vi "trigger.vi"(8 "error in (no error)":errorcluster, 11 "handle":u32) -> (0 "error out":errorcluster, 2 "function return":i32, 3 "handle out":i32)   [LabVIEW 2017, in "buddy.lvlib"]
doc: "EXPORT int buddy_trigger(hid_device *handle);"
uses:
  buddy.lvlib
  buddy_x64.dll
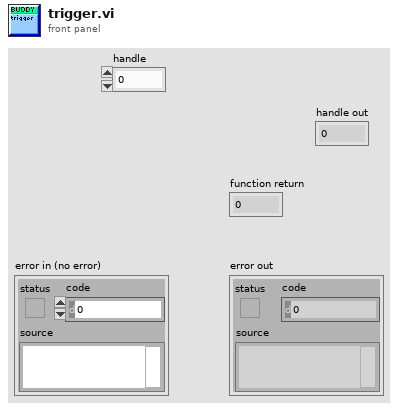
[diagram p1: front panel]
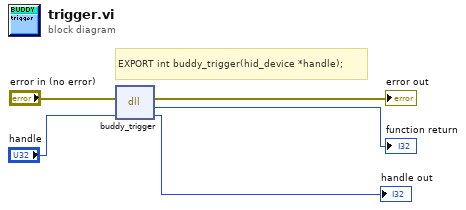
[diagram p0: block diagram]
diagram:
  # "EXPORT int buddy_trigger(hid_device *handle);"
  n1 = dll-call lib="C:/Users/shraken/shraken_code/usbhid_buddy/lib/libbuddy/bindings/labview/utility_vi/buddy_x64.dll" fn="buddy_trigger"(error in="error in (no error)", "handle"="handle") -> (error out=→"error out":errorcluster, "return type"=→"function return":i32, "handle"=→"handle out":u32)  [unwired: 2 in, 1 out]
